vi "Set VI param.vi"(4 "log path":path, 6 "host FIFO depth":u32=256000 format="%.3p", 7 "Time Target (s)":dbl=1.0 caption="Time target(s)", 8 "Error In":errorcluster caption="エラー入力", 9 "number of samples":u32=256000 caption="Number of Samples", 10 "sample rate":dbl=200000000.0 caption="Sample Rate" format="%#.3pS/s", 11 "VI refnum":refnum<vi>) -> (0 "Error Out":errorcluster caption="エラー出力", 3 "リファレンス出力":refnum<vi>)   [LabVIEW 2018]
uses:
  Host/SubVIs/Start Trigger.ctl
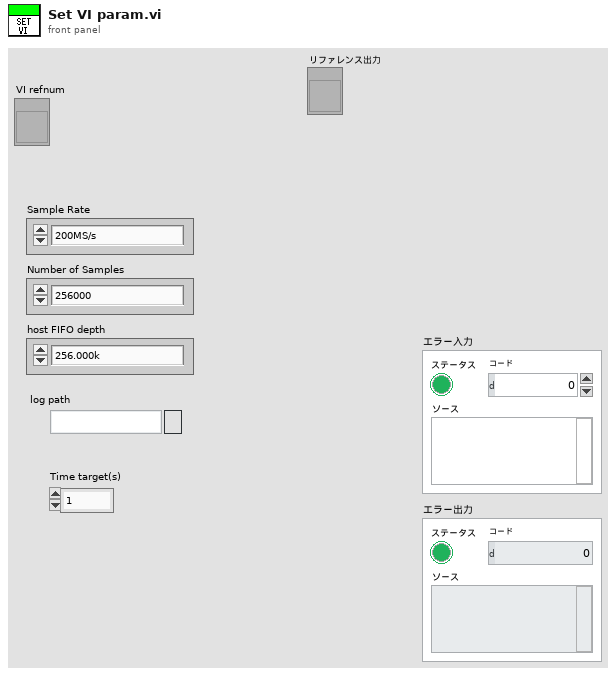
[diagram p1: front panel]
types:
  T1 = typedef "Start Trigger.ctl" = enum8{"Software", "Digital Edge", "Rx Start Trigger", "Tx Start Trigger", "Immediate", "Future Time Event"}
  T2 = cluster{"rf enable 0":bool, "rf config 0":cluster{"antenna":string, "frequency":dbl, "lo frequency":dbl, "level":dbl}, "rf enable 1":bool, "rf config 1":cluster{"antenna":string, "frequency":dbl, "lo frequency":dbl, "level":dbl}, "transfer mode":enum16{"Finite", "Continuous"}, "sample rate":dbl, "number of samples":u32, "start trigger":T1}
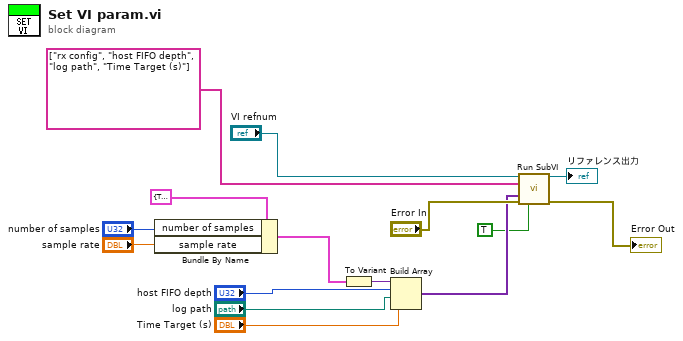
[diagram p0: block diagram]
diagram:
  n1 = Bundle By Name(cluster=T2 {"rf enable 0"=TRUE, "rf config 0"={"antenna"="RX2", "frequency"=2000000000.0, "lo frequency"=-1.0, "level"=0.0}, "rf enable 1"=FALSE, "rf config 1"={"antenna"="RX2", "frequency"=2000000000.0, "lo frequency"=-1.0, "level"=0.0}, "transfer mode"=enum."Continuous", "sample rate"=200000000.0, "number of samples"=256000, "start trigger"=enum."Immediate"} ("rx config"), "number of samples"="number of samples", "sample rate"="sample rate") -> (w5:T2)
  n2 = To Variant(anything=w5) -> (Variant=w4:variant)
  n3 = Build Array(w4, "host FIFO depth", "log path", "Time Target (s)") -> (w11:variant[])
  n4 = call "Run SubVI.vi"("VIリファレンス"="VI refnum", "Value Ctl Names"=string[] ["rx config", "host FIFO depth", "log path", "Time Target (s)"], "Values"=w11, "error in (no error)"="Error In", "終了まで待機 (F)"=TRUE) -> ("リファレンス出力"=→"リファレンス出力":refnum<vi>, "error out"=→"Error Out":errorcluster)  [unwired: 9 in]
